vi "HEWH Removed Unnecessary Data.vi"(8 "Error In":errorcluster, 10 "Data With Headers":string[][](array[string])) -> (0 "Error Out":errorcluster, 2 "Stat Data Output":string[][](array[string]), 3 "Draw Stats Out":dbl[](array[numeric]))   [LabVIEW 2019]
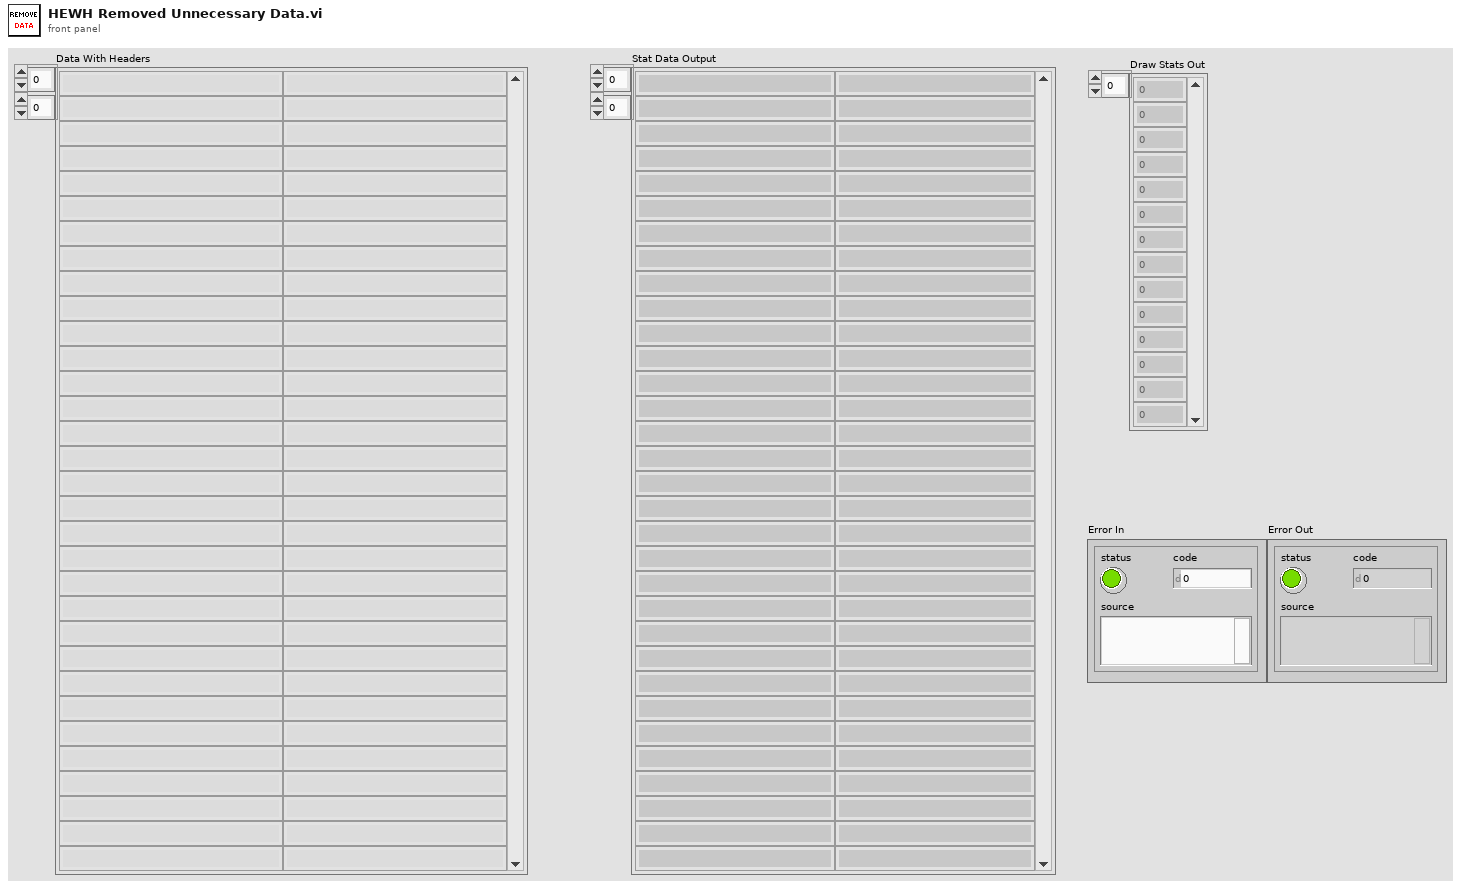
[diagram p1: front panel]
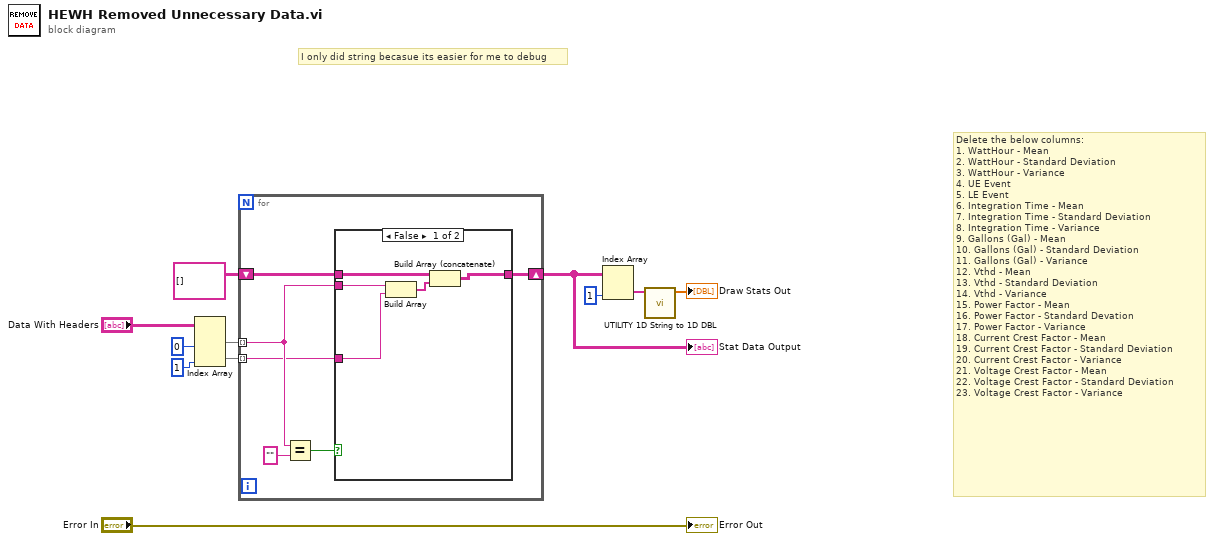
[diagram p0: block diagram]
diagram:
  # "I only did string becasue its easier for me to debug"
  # "Delete the below columns:\n1. WattHour - Mean\n2. WattHour - Standard Deviation\n3. WattHour - Variance\n4. UE Event\n5. LE Event\n6. Integration Time - Mean\n7. Integration Time - Standard Deviation\n8. Integration Time - Variance\n9. Gallons (Gal) - Mean\n10. Gallons (Gal) - Standard Deviation\n11. Gallons (Gal) - Variance \n12. Vthd - Mean\n13. Vthd - Standard Deviation\n14. Vthd - Variance\n15. Power Factor - Mean\n16. Power Factor - Standard Devation\n17. Power Factor - Variance\n18. Current Crest Factor - Mean\n19. Current Crest Factor - Standard Deviation\n20. Current Crest Factor - Variance\n21. Voltage Crest Factor - Mean\n22. Voltage Crest Factor - Standard Deviation\n23. Voltage Crest Factor - Variance"
  n1 = Index Array(array="Data With Headers", index (col) #1=0 ("disabled index (col)"), index (col) #2=1 ("index (col)")) -> (element #1=w9:string[], element #2=w7:string[])  [unwired: 2 in]
  n2 = for {
    tunnel: w9 -> [w15] mode=indexing
    tunnel: w7 -> [w14] mode=indexing
    shift-right: [w12] -> w5
    shift-left: string[][] [] -> [w13]
    n3 = Equal?(x=w15, y="") -> (x = y?=w16:bool)
    n4 = case shown="False" w16 {
      tunnel: w15 -> [w22 _]
      tunnel: w14 -> [w21 _]
      tunnel: w13 -> [w20 w23]
      tunnel: [w18 w23] -> w12
      frame False {
        n5 = Build Array(w22, w21) -> (w19:string[])
        n6 = Build Array (concatenate)(w20, w19) -> (w18:string[][])
      }
      frame True {
      }
    }
  }
  "Stat Data Output" <- w5
  n7 = Index Array(array=w5, index (col)=1 ("disabled index (col)")) -> (element=w3:string[])  [unwired: 1 in]
  n8 = call "UTILITY 1D String to 1D DBL.vi"("Save Data"=w3) -> ("DBL"=→"Draw Stats Out":dbl[])  [unwired: 10 in]
  "Error Out" <- "Error In"
